vi "memory_sim.vi"(9 "data in":u32, 10 "t-read;fwrite":bool, 11 "index":u32) -> (1 "Array":u32[](array[numeric]), 3 "element out":u32)   [LabVIEW 2021]
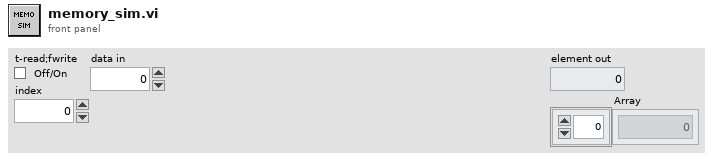
[diagram p1: front panel]
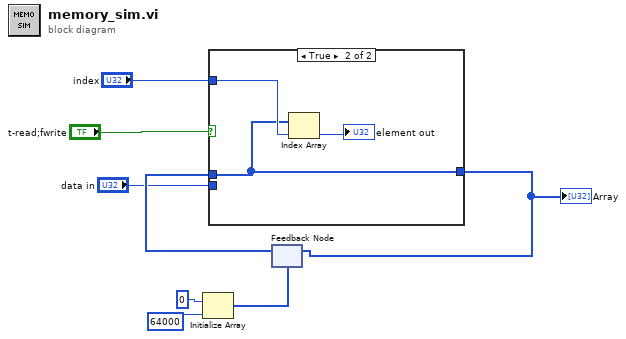
[diagram p0: block diagram]
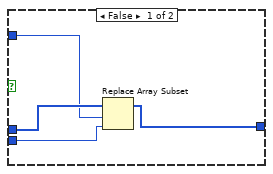
[diagram p2: hidden frame]
diagram:
  n1 = Initialize Array(u32 0, 64000 ("dimension size")) -> (w6:u32[])
  n2 = feedback #1(w6) -> (w5:u32[])
  n3 = case shown="False" "t-read;fwrite" {
    tunnel: w5 -> [w12 w14]
    tunnel: "index" -> [w10 w15]
    tunnel: [w11 w14] -> w2
    tunnel: "data in" -> [w9 _]
    frame False {
      n4 = Replace Array Subset(array=w12, new element=w9, index=w10) -> (w11:u32[])
    }
    frame True {
      n5 = Index Array(array=w14, index=w15) -> (element=→"element out":u32)
    }
  }
  "Array" <- w2
  n6 = feedback-in #1(w2) -> ()
